vi "Get Cache System Actions.vi"(8 "error in (no error)":errorcluster, 11 "TLB' Error Handler in":refnum<class "TLB` Error Handler.lvclass">) -> (0 "error out":errorcluster, 2 "Cache System Actions":string[](array[string]), 3 "TLB' Error Handler out":refnum<class "TLB` Error Handler.lvclass">)   [LabVIEW 2018, in "Springboard TLB`.lvlib" / "TLB` Error Handler.lvclass"]
uses:
  TLB` Error Handler.lvclass
  TLB` Error Handler.lvclass/TLB` Error Handler.ctl
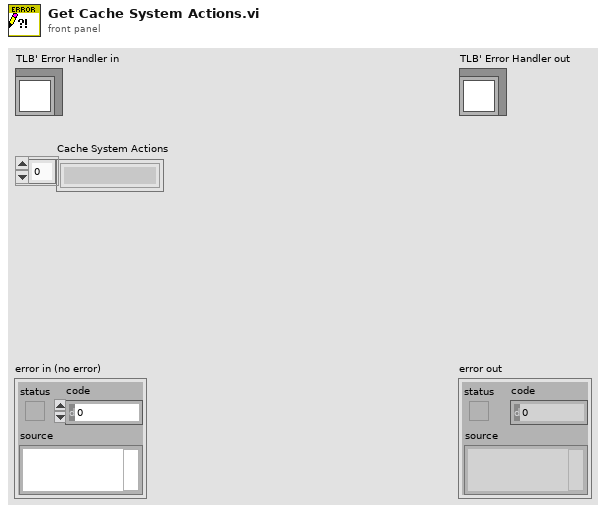
[diagram p1: front panel]
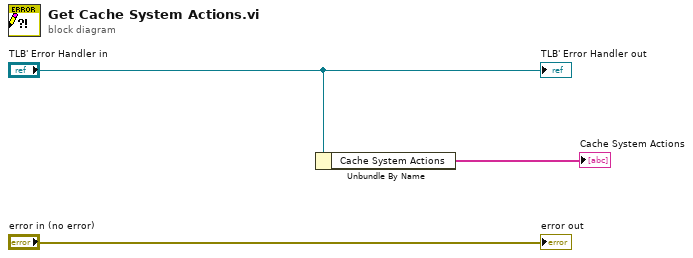
[diagram p0: block diagram]
diagram:
  n1 = Unbundle By Name("TLB' Error Handler in") -> ("Cache System Actions"=→"Cache System Actions":string[])
  "error out" <- "error in (no error)"
  "TLB' Error Handler out" <- "TLB' Error Handler in"
